vi "write_fifo.vi"(7 "pixel-to-host\n mode":T1, 8 "FIFO overflow in":bool, 10 "block index in":i32, 11 "values to be written":T2) -> (0 "FIFO overflow out":bool, 2 "block index out":i32, 3 "channels out":T2)   [LabVIEW 2010]
uses:
  FPGA_Typedefs/channels_array.ctl
  FPGA_Typedefs/pixel_to_host_enum.ctl
  <vilib>/rvi/DataTransferAndStorage/Container/XNode/niFpgaContainer.xnode
  <vilib>/rvi/DataTransferAndStorage/Container/Common/niFpgaContainerMethod.ctl
  <vilib>/rvi/DataTransferAndStorage/Container/Common/niFpgaTransferTypeControl.ctl
  <vilib>/rvi/interface/RandomDataEmulation/nirviRandomDataFPGAFIFO.vi
  <vilib>/rvi/interface/RandomDataEmulation/niFpgaRandomDataHandleErrors.vi
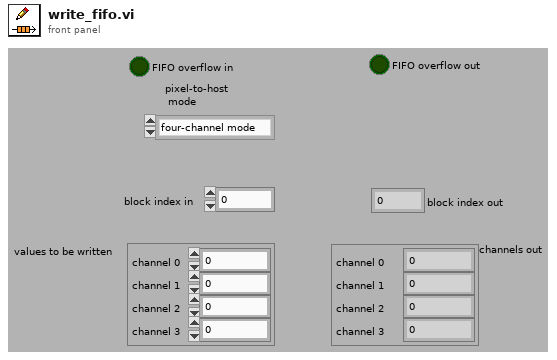
[diagram p1: front panel]
types:
  T1 = typedef "pixel_to_host_enum.ctl" = enum16{"four-channel mode", "two-channel mode"}
  T2 = typedef "channels_array.ctl" = cluster{"channel 0":u32, "channel 1":u32, "channel 2":u32, "channel 3":u32}
  T3 = typedef "niFpgaContainerMethod.ctl" = enum16{"<none>", "write", "read", "clear", "getNumberOfElementsToWrite", "getNumberOfElementsToRead", "enable", "disable", "flushAndDisable", "getStreamState", "readA", "readB", "dramWrite", "dramWriteWithByteEnables", "dramRequestData", "dramRetrieveData"}
  T4 = typedef "niFpgaTransferTypeControl.ctl" = enum16{"Target-Scoped", "Host to Target - DMA", "Target to Host - DMA", "Peer to Peer Reader", "Peer to Peer Writer", "Bidirectional"}
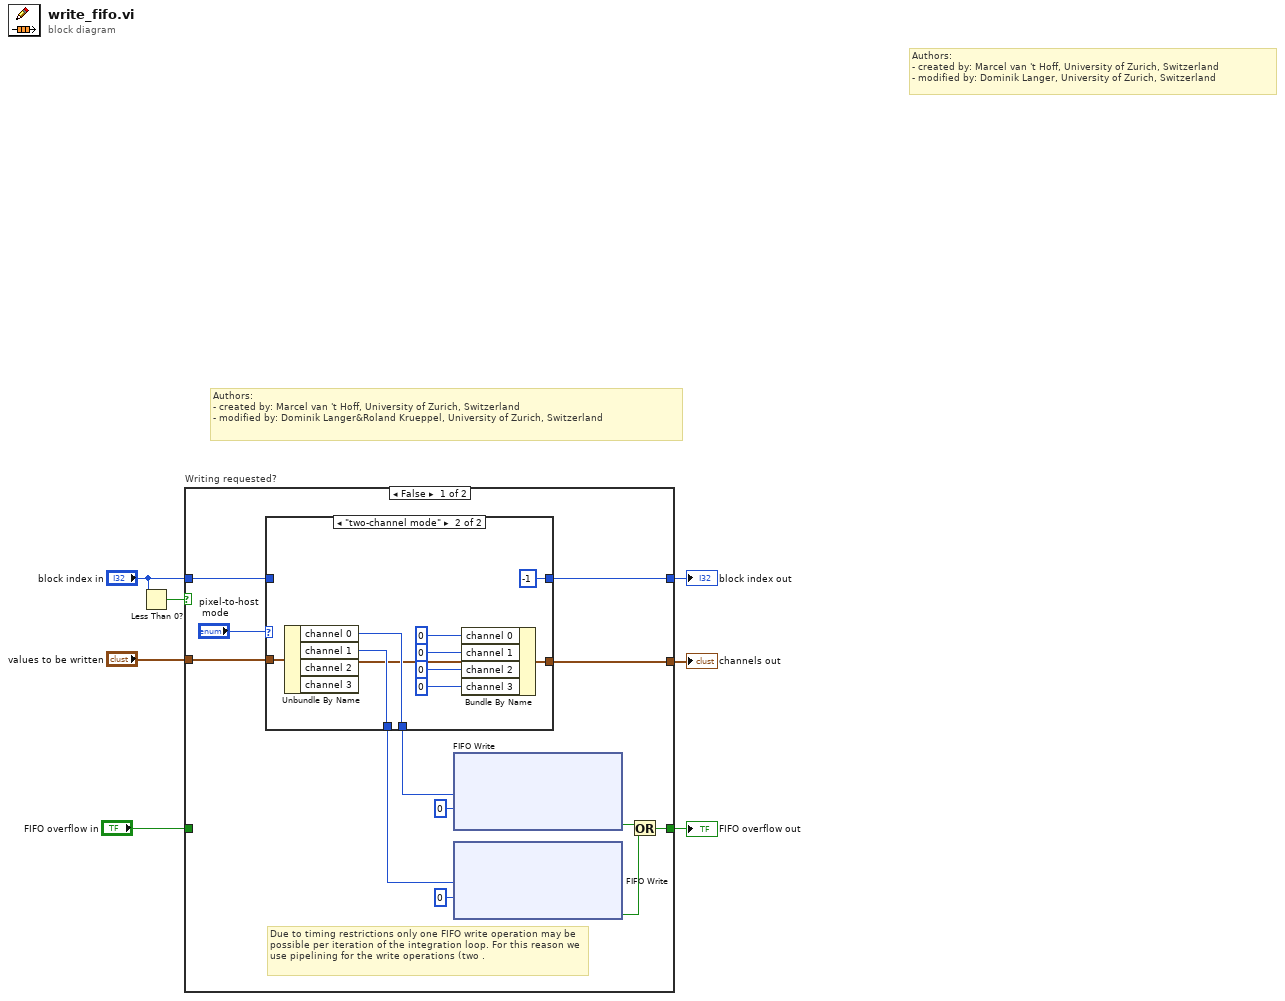
[diagram p0: block diagram]
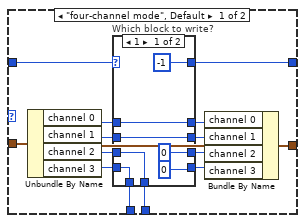
[diagram p2: hidden frame]
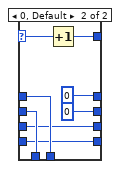
[diagram p3: hidden frame]
diagram:
  # "Authors: \n- created by: Marcel van 't Hoff, University of Zurich, Switzerland\n- modified by: Dominik Langer&Roland Krueppel, University of Zurich, Switzerland"
  # "Authors: \n- created by: Marcel van 't Hoff, University of Zurich, Switzerland\n- modified by: Dominik Langer, University of Zurich, Switzerland"
  n1 = Less Than 0?(x="block index in") -> (x < 0?=w3:bool)
  n2 = case "Writing requested?" shown="False" w3 {
    tunnel: [w14 w115] -> w4
    tunnel: [w11 w116] -> w7
    tunnel: "block index in" -> [w13 w116]
    tunnel: "values to be written" -> [w12 w115]
    tunnel: "FIFO overflow in" -> [_ w114]
    tunnel: [w15 w114] -> w1
    frame False {
      # "Due to timing restrictions only one FIFO write operation may be possible per iteration of the integration loop. For this reason we use pipelining for the write operations (two ."
      n3 = case shown="\"two-channel mode\"" "pixel-to-host\n mode" {
        tunnel: [w23 w51] -> w14
        tunnel: w13 -> [w20 _]
        tunnel: w12 -> [w25 w50]
        tunnel: [w24 -1 ("block index in")] -> w11
        tunnel: [w22 w56] -> w8
        tunnel: [w21 w57] -> w9
        frame "four-channel mode", Default {
          n4 = Unbundle By Name(w25) -> ("channel 0"=w26:u32, "channel 1"=w27:u32, "channel 2"=w28:u32, "channel 3"=w29:u32)
          n5 = case "Which block to write?" shown="1" w20 {
            selector: w20 -> [_ w41]
            tunnel: [w40 w48] -> w21
            tunnel: w26 -> [w38 w48]
            tunnel: [w39 w47] -> w22
            tunnel: w27 -> [w37 w47]
            tunnel: w28 -> [w40 w46]
            tunnel: w29 -> [w39 w45]
            tunnel: [u32 0 ("channel 2") w46] -> w31
            tunnel: [u32 0 ("channel 3") w45] -> w30
            tunnel: [w38 u32 0 ("channel 0")] -> w32
            tunnel: [w37 u32 0 ("channel 1")] -> w33
            tunnel: [-1 ("block index in") w42] -> w24
            frame 1 {
            }
            frame 0, Default {
              n6 = Increment(x=w41) -> (x+1=w42:i32)
            }
          }
          n7 = Bundle By Name(cluster=w25, "channel 0"=w32, "channel 1"=w33, "channel 2"=w31, "channel 3"=w30) -> (w23:T2)
        }
        frame "two-channel mode" {
          n8 = Unbundle By Name(w50) -> ("channel 0"=w57:u32, "channel 1"=w56:u32)  [unwired: 2 out]
          n9 = Bundle By Name(cluster=w50, "channel 0"=u32 0, "channel 1"=u32 0, "channel 2"=u32 0 ("channel 0"), "channel 3"=u32 0 ("channel 1")) -> (w51:T2)
        }
      }
      n10 = xnode ("FIFO Write")("Element"=w9, "Timeout"=0) -> ("Timed Out?"=w16:bool)  [unwired: 1 in, 1 out]
      n11 = xnode ("FIFO Write")("Element"=w8, "Timeout"=0) -> ("Timed Out?"=w17:bool)  [unwired: 1 in, 1 out]
      n12 = Or(x=w16, y=w17) -> (x .or. y?=w15:bool)
    }
    frame True {
    }
  }
  "channels out" <- w4
  "block index out" <- w7
  "FIFO overflow out" <- w1
